vi "3D-sub2Array.vi"(10 "X":i32[](array[numeric]), 11 "pic z value":dbl[][](array[numeric])) -> (1 "最大值":dbl, 2 "行值":i32, 3 "列值":i32)   [LabVIEW 2015]
panel:
  out "列":i32
  out "行":i32
  out "数组":dbl[][](array[numeric])
  out "Y Distance":i32
  out "X Distance":i32
  out "Bottom":i32
  out "Right":i32
  out "Top":i32
  out "Left":i32
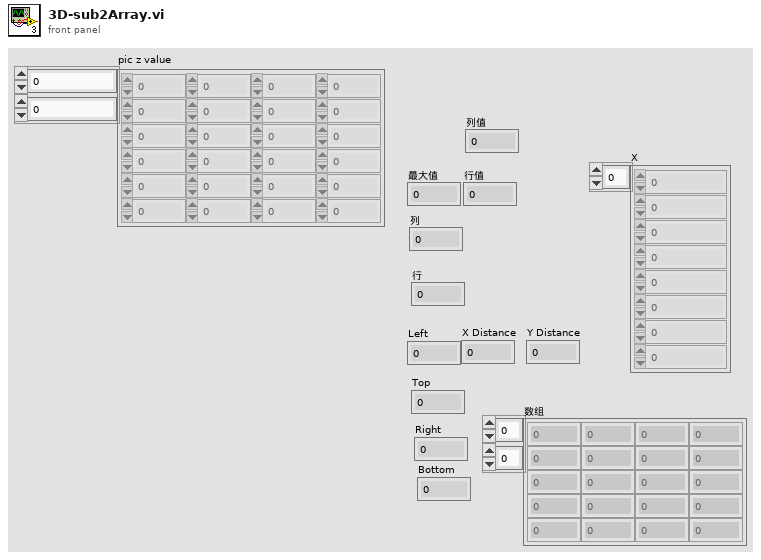
[diagram p1: front panel]
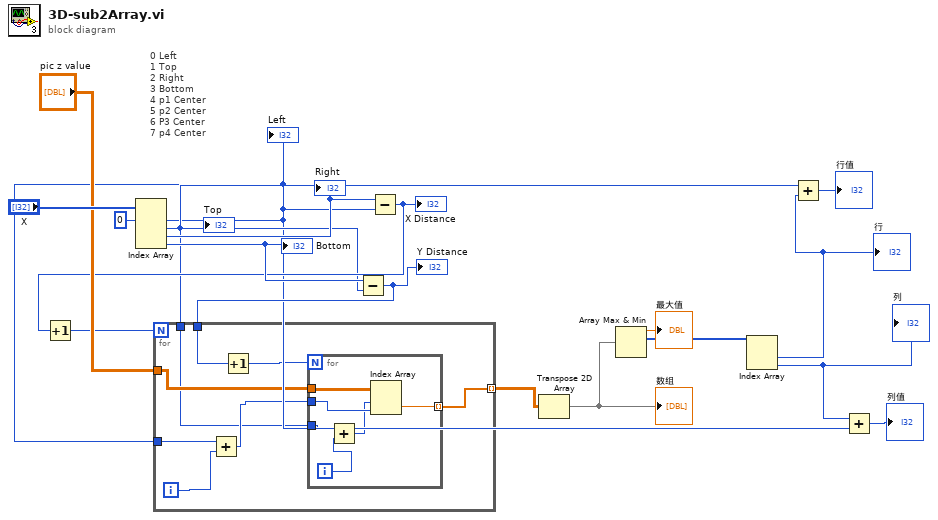
[diagram p0: block diagram]
diagram:
  # "0 Left\n1 Top\n2 Right\n3 Bottom\n4 p1 Center\n5 p2 Center\n6 P3 Center\n7 p4 Center"
  n1 = Index Array(array="X", index #1=0 ("索引")) -> (element #1=w2:i32, element #2=w5:i32, element #3=w16:i32, element #4=w15:i32)  [unwired: 3 in]
  "Left" <- w2
  "Top" <- w5
  "Right" <- w16
  "Bottom" <- w15
  n2 = Subtract(x=w15, y=w5) -> (x-y=w11:i32)
  "Y Distance" <- w11
  n3 = Subtract(x=w16, y=w2) -> (x-y=w13:i32)
  "X Distance" <- w13
  n4 = Increment(x=w13) -> (x+1=w12:i32)
  n5 = for {
    N: w12 -> [_]
    tunnel: "pic z value" -> [w26]
    tunnel: w11 -> [w23]
    tunnel: [w25] -> w10 mode=indexing
    tunnel: w2 -> [w21]
    tunnel: w5 -> [w19]
    i -> [w24]
    n6 = Add(x=w21, y=w24) -> (x+y=w20:i32)
    n7 = Increment(x=w23) -> (x+1=w22:i32)
    n8 = for {
      N: w22 -> [_]
      tunnel: w26 -> [w32]
      tunnel: w20 -> [w31]
      tunnel: [w30] -> w25 mode=indexing
      tunnel: w19 -> [w28]
      i -> [w29]
      n9 = Add(x=w28, y=w29) -> (x+y=w27:i32)
      n10 = Index Array(array=w32, index (row)=w27, index (col)=w31) -> (element=w30:dbl)
    }
  }
  n11 = Transpose 2D Array(2D array=w10) -> (transposed array=w9:dbl[][])
  "数组" <- w9
  n12 = Array Max & Min(array=w9) -> (max value=→"最大值":dbl, max index (indices)=w7:i32[])  [unwired: 2 out]
  n13 = Index Array(array=w7) -> (element #1=w6:i32, element #2=w3:i32)  [unwired: 2 in]
  "行" <- w6
  "列" <- w3
  n14 = Add(x=w5, y=w6) -> (x+y=→"行值":i32)
  n15 = Add(x=w3, y=w2) -> (x+y=→"列值":i32)
